vi "VerifyString.vi"(4 "Expected String":string, 5 "String To Verify":string) -> (2 "Are Strings Equal?":bool)   [LabVIEW 2013]
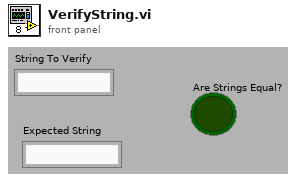
[diagram p1: front panel]
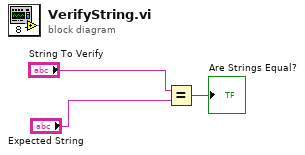
[diagram p0: block diagram]
diagram:
  n1 = Equal?(x="String To Verify", y="Expected String") -> (x = y?=→"Are Strings Equal?":bool)
